vi "First_Num_from_String.vi"(1 "string":string) -> (0 "number":dbl)   [LabVIEW 2020]
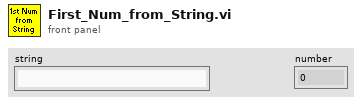
[diagram p1: front panel]
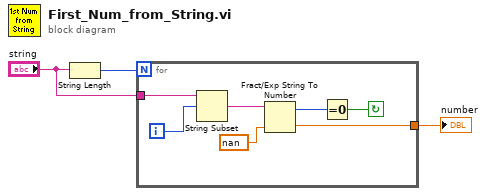
[diagram p0: block diagram]
diagram:
  n1 = String Length(string="string") -> (length=w2:i32)
  n2 = for {
    N: w2 -> [_]
    tunnel: "string" -> [w9]
    tunnel: [w4] -> w3
    i -> [w10]
    stop <- w5 continue-if-true
    n3 = String Subset(string=w9, offset (0)=w10) -> (substring=w8:string)  [unwired: 1 in]
    n4 = Fract/Exp String To Number(string=w8, default (0 dbl)=nan ("default (0 DBL)")) -> (offset past number=w6:i32, number=w4:dbl)  [unwired: 2 in]
    n5 = Equal To 0?(x=w6) -> (x = 0?=w5:bool)
  }
  "number" <- w3
